vi "Pack for gRPC.vi"(8 "error in":errorcluster, 9 "configuration / results":enum16{"Configuration", "Results"}(ring), 10 "data value":variant, 11 "measurement in":refnum<class "Continuous Counting Measurement.lvclass">) -> (0 "error out":errorcluster, 2 "any":T1, 3 "measurement out":refnum<class "Continuous Counting Measurement.lvclass">)   [LabVIEW 2021, in "MeasurementServerTests.lvlib" / "Measurement Service Tests.lvlib" / "Continuous Counting Measurement.lvclass"]
uses:
  Continuous Counting Measurement.lvclass
  <vilib>/gRPC/LabVIEW gRPC Library/Shared/Any.ctl
  C:/Dev/github/ni/measurementlink-labview/Source/Runtime/Measurements/Measurement Plugin Service/Measurement Plugin Service.lvclass
  Measurement Configuration.ctl
  Measurement Results.ctl
  59b0e5df-407b-4a5d-9477-f9caddb4022e.vi
  cefe5da3-be5c-4446-8480-824a8bbdf22b.vi
  <vilib>/gRPC/LabVIEW gRPC Library/Server API/Translate Protobuf Error.vi
  <vilib>/AdvancedString/1D String Array to Delimited String.vi
  <vilib>/gRPC/LabVIEW gRPC Library/Server API/Server/Get Server DLL Path.vi
  Runtime/Measurements/Measurement Plugin Service/Measurement Plugin Service.lvclass
  <vilib>/gRPC/LabVIEW gRPC Library/grpc-lvsupport-release.lvlib
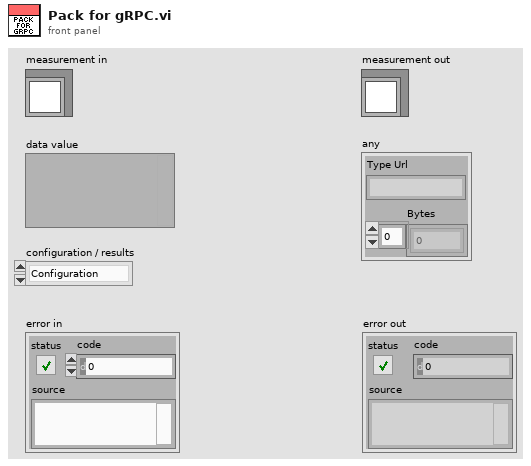
[diagram p1: front panel]
types:
  T1 = typedef "grpc-lvsupport-release.lvlib/Any.ctl" = cluster{"Type Url":string, "Bytes":u8[]}
  T2 = typedef "grpc-lvsupport-release.lvlib/grpcId.ctl" = u64
  T3 = typedef "MeasurementServerTests.lvlib/Measurement Service Tests.lvlib/Continuous Counting Measurement.lvclass/Measurement Configuration.ctl" = cluster{"ms update interval":u32}
  T4 = typedef "MeasurementServerTests.lvlib/Measurement Service Tests.lvlib/Continuous Counting Measurement.lvclass/Measurement Results.ctl" = cluster{"current count":i64}
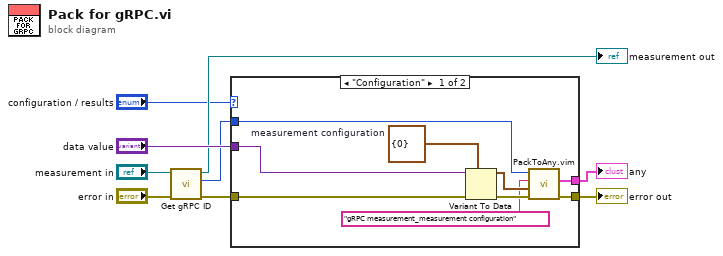
[diagram p0: block diagram]
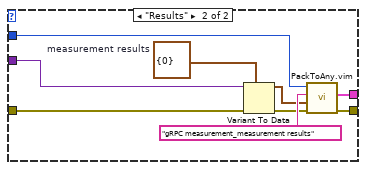
[diagram p2: hidden frame]
diagram:
  n1 = call "Get gRPC ID.vi"("error in"="error in", "measurement plugin service in"="measurement in") -> ("error out"=w5:errorcluster, "gRPC ID"=w2:T2, "measurement plugin service out"=→"measurement out":refnum<class "Continuous Counting Measurement.lvclass">)  [unwired: 7 in]
  n2 = case shown="\"Configuration\"" "configuration / results" {
    tunnel: w5 -> [w18 w27]
    tunnel: "data value" -> [w17 w26]
    tunnel: w2 -> [w14 w23]
    tunnel: [w16 w25] -> w9
    tunnel: [w15 w24] -> w8
    frame "Configuration" {
      w10 = T3 {"ms update interval"=0}  # measurement configuration
      n3 = Variant To Data(error in=w18, type=w10, Variant=w17) -> (data=w13:T3, error out=w12:errorcluster)
      n4 = call "PackToAny.vim"("error in"=w12, "Data To Pack"=w13, "Message Type"="gRPC measurement_measurement configuration", "gRPCid in"=w14) -> ("error out"=w16:errorcluster, "Any"=w15:T1)  [unwired: 5 in, 1 out]
    }
    frame "Results" {
      w19 = T4 {"current count"=0}  # measurement results
      n5 = Variant To Data(error in=w27, type=w19, Variant=w26) -> (data=w21:T4, error out=w20:errorcluster)
      n6 = call "PackToAny.vim"("error in"=w20, "Data To Pack"=w21, "Message Type"="gRPC measurement_measurement results", "gRPCid in"=w23) -> ("error out"=w25:errorcluster, "Any"=w24:T1)  [unwired: 5 in, 1 out]
    }
  }
  "error out" <- w9
  "any" <- w8
